vi "DE_Penalize with Equality Constraints.vi"(10 "Equality Constraints":dbl[](array[numeric]), 11 "Objective Functions In":dbl[](array[numeric])) -> (3 "Objective Functions Out":dbl[](array[numeric]))   [LabVIEW 2017, in "NI_AAL_GlobalOptimization.lvlib"]
uses:
  <vilib>/gmath/NI_AAL_GlobalOptimization.lvlib
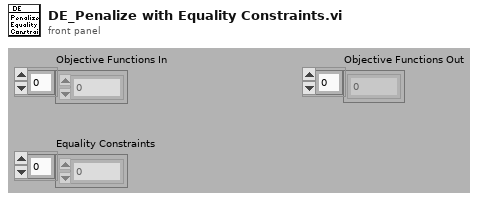
[diagram p1: front panel]
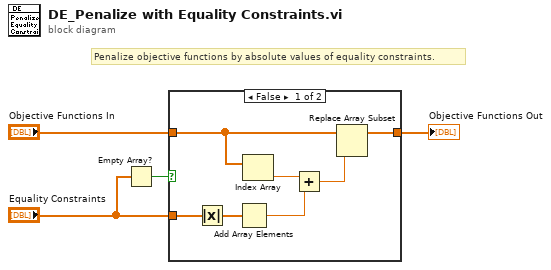
[diagram p0: block diagram]
diagram:
  # "Penalize objective functions by absolute values of equality constraints."
  n1 = Empty Array?(array="Equality Constraints") -> (empty?=w4:bool)
  n2 = case shown="False" w4 {
    tunnel: "Equality Constraints" -> [w11 _]
    tunnel: "Objective Functions In" -> [w7 w12]
    tunnel: [w5 w12] -> w1
    frame False {
      n3 = Absolute Value(x=w11) -> (abs(x)=w10:dbl[])
      n4 = Add Array Elements(numeric array=w10) -> (sum=w8:dbl)
      n5 = Index Array(array=w7) -> (element=w9:dbl)  [unwired: 1 in]
      n6 = Add(x=w9, y=w8) -> (x+y=w6:dbl)
      n7 = Replace Array Subset(array=w7, new element=w6) -> (w5:dbl[])  [unwired: 1 in]
    }
    frame True {
    }
  }
  "Objective Functions Out" <- w1
